vi "Get 1 Trace from SCADA.vi"(9 "Numeric":i32, 10 "seconds since 1Jan1904":timestamp, 11 "Tag":string) -> (3 "Cluster":cluster{timestamp[], dbl[]})   [LabVIEW 2019]
uses:
  <vilib>/httpClient/LabVIEWHTTPClient.lvlib
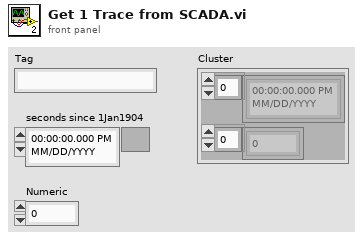
[diagram p1: front panel]
types:
  T1 = cluster{"firstTimestamp":string, "sampleInterval":i32, "data":dbl[]}
  T2 = typedef "LabVIEWHTTPClient.lvlib/ClientHandle.ctl" = refnum<k1>
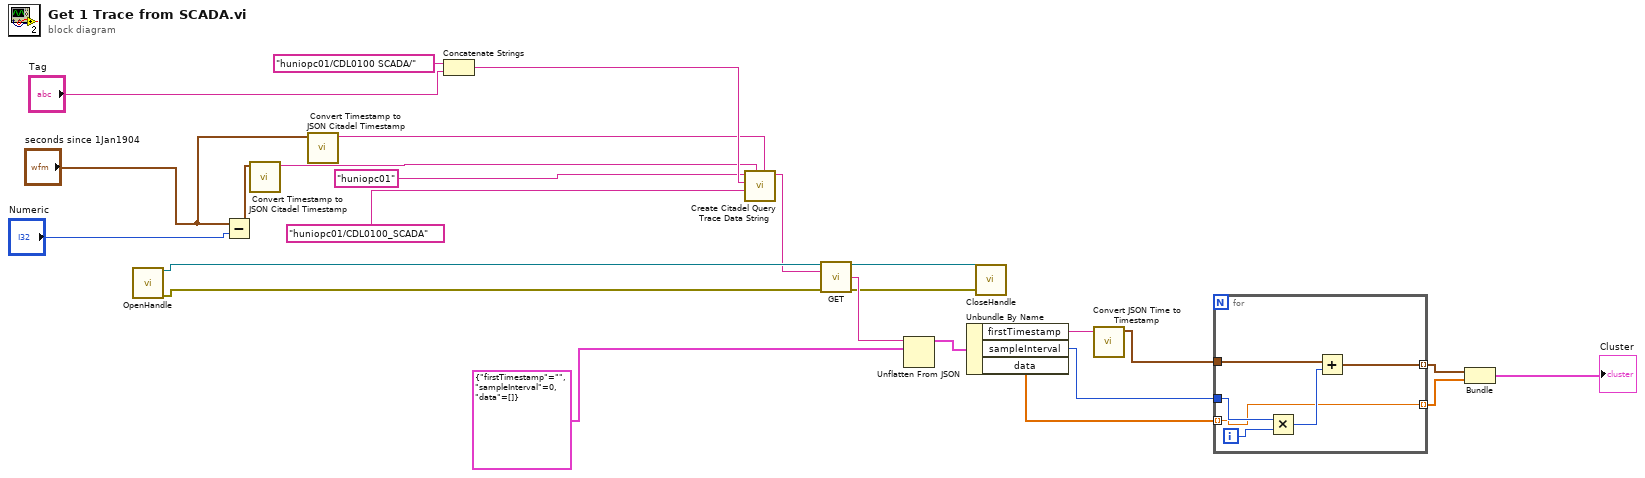
[diagram p0: block diagram]
diagram:
  n1 = call <vilib>:"OpenHandle.vi"() -> ("client handle out"=w12:T2, "error out"=w13:errorcluster)  [unwired: 14 in]
  n2 = Subtract(x="seconds since 1Jan1904", y="Numeric") -> (x-y=w2:timestamp)
  n3 = call "Convert Timestamp to JSON Citadel Timestamp.vi"("time stamp"=w2) -> ("Citadel date/time string"=w5:string)  [unwired: 10 in]
  n4 = call "Convert Timestamp to JSON Citadel Timestamp.vi"("time stamp"="seconds since 1Jan1904") -> ("Citadel date/time string"=w4:string)  [unwired: 10 in]
  n5 = Concatenate Strings("huniopc01/CDL0100 SCADA/" ("string"), "Tag") -> (w10:string)
  n6 = call "Create Citadel Query Trace Data String.vi"("End Time String"=w4, "Start Time String"=w5, "db Path"="huniopc01/CDL0100_SCADA", "Trace Name"=w10, "Server"="huniopc01") -> ("GET string"=w11:string)  [unwired: 5 in, 1 out]
  n7 = call <vilib>:"GET.vi"("client handle"=w12, "url"=w11, "error in (no error)"=w13) -> ("client handle out"=w15:T2, "body"=w16:string, "error out"=w14:errorcluster)  [unwired: 9 in, 1 out]
  n8 = Unflatten From JSON(JSON string=w16, type and defaults=T1 {"firstTimestamp"="", "sampleInterval"=0, "data"=[]}) -> (value=w18:T1)  [unwired: 5 in, 1 out]
  n9 = Unbundle By Name(w18) -> ("firstTimestamp"=w19:string, "sampleInterval"=w21:i32, "data"=w22:dbl[])
  n10 = call <vilib>:"CloseHandle.vi"("client handle"=w15, "error in (no error)"=w14) -> ()  [unwired: 13 in, 1 out]
  n11 = call "Convert JSON Time to Timestamp.vi"("JSON Citadel Time string"=w19) -> ("time stamp"=w20:timestamp)  [unwired: 10 in]
  n12 = for {
    tunnel: w22 -> [w26] mode=indexing
    tunnel: w21 -> [w31]
    tunnel: w20 -> [w29]
    tunnel: [w27] -> w23 mode=indexing
    tunnel: [w26] -> w24 mode=indexing
    i -> [w30]
    n13 = Multiply(x=w31, y=w30) -> (x*y=w28:i32)
    n14 = Add(x=w29, y=w28) -> (x+y=w27:timestamp)
  }
  n15 = Bundle(w23, w24) -> (→"Cluster":cluster{timestamp[], dbl[]})  [unwired: 1 in]
